vi "1.5.12-GainMultiplyNoServer.vi"(0 "Gain Exponent":i8, 5 "Gain":fxp<+/-,18,1> format="%.18g", 9 "Input":fxp<+/-,18,1> format="%.18g") -> (3 "Result is Good":bool, 8 "Output":fxp<+/-,18,1> format="%.18g")   [LabVIEW 2010]
uses:
  <vilib>/rvi/FXPMathLib/FxpMul/XNode/nifxpmath_Multiplier.xnode
  <vilib>/rvi/FXPMathLib/FxpMul/subVIs/nifxpmath_Mul_SimConfig.ctl
  <vilib>/fxp/LVFixedPointQuantizationPolicyTypeDef.ctl
  <vilib>/fxp/LVFixedPointOverflowPolicyTypeDef.ctl
  <vilib>/rvi/FXPMathLib/FxpMul/simVIs/DllFxpMulTemp_sub.vi
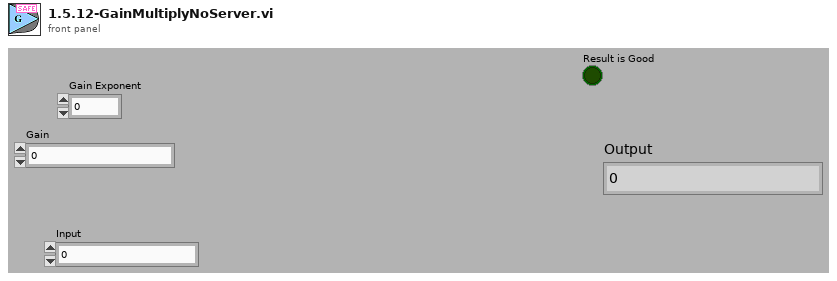
[diagram p1: front panel]
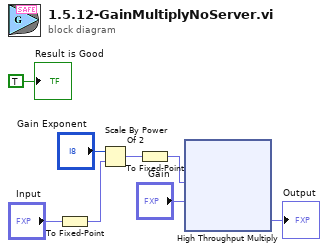
[diagram p0: block diagram]
diagram:
  n1 = To Fixed-Point(number="Input") -> (fixed-point=w5:fxp<+/-,54,18>)  [unwired: 1 in]
  n2 = Scale By Power Of 2(n="Gain Exponent", x=w5) -> (x*2^n=w6:fxp<+/-,54,18>)
  n3 = To Fixed-Point(number=w6) -> (fixed-point=w4:fxp<+/-,18,1>)  [unwired: 1 in]
  n4 = xnode "High Throughput Multiply"("x"=w4, "y"="Gain") -> ("x*y"=→"Output":fxp<+/-,18,1>)
  "Result is Good" <- TRUE ("Result is Good")
